vi "InsertDBNew.vi"(9 "String":string, 11 "Entity":string) -> (0 "error out":errorcluster)   [LabVIEW 2012]
uses:
  Global1.vi
  <vilib>/addons/database/Connection.llb/DB Tools Open Connec (Path).vi
  <vilib>/Utility/file.llb/Read From Spreadsheet File (string).vi
  <vilib>/Utility/file.llb/Read From Spreadsheet File (I64).vi
  <vilib>/addons/database/Connection.llb/Conn Execute.vi
  <vilib>/addons/database/Recordset.llb/Rec Fetch Integer Data (R).vi
  <vilib>/addons/database/Recordset.llb/Rec Destroy - Connection.vi
  <vilib>/regexp/Match Regular Expression.xnode
  <vilib>/addons/database/NI_Database_API.lvlib
panel:
  out "output cluster":T1
  out "PathM100":path=path "c:/m100"
  out "appended path":path
  out "concatenated string":string
  out "file or folder exists?":bool
  out "element 7":string
  out "before substring 9":string
  in  "input cluster":T1
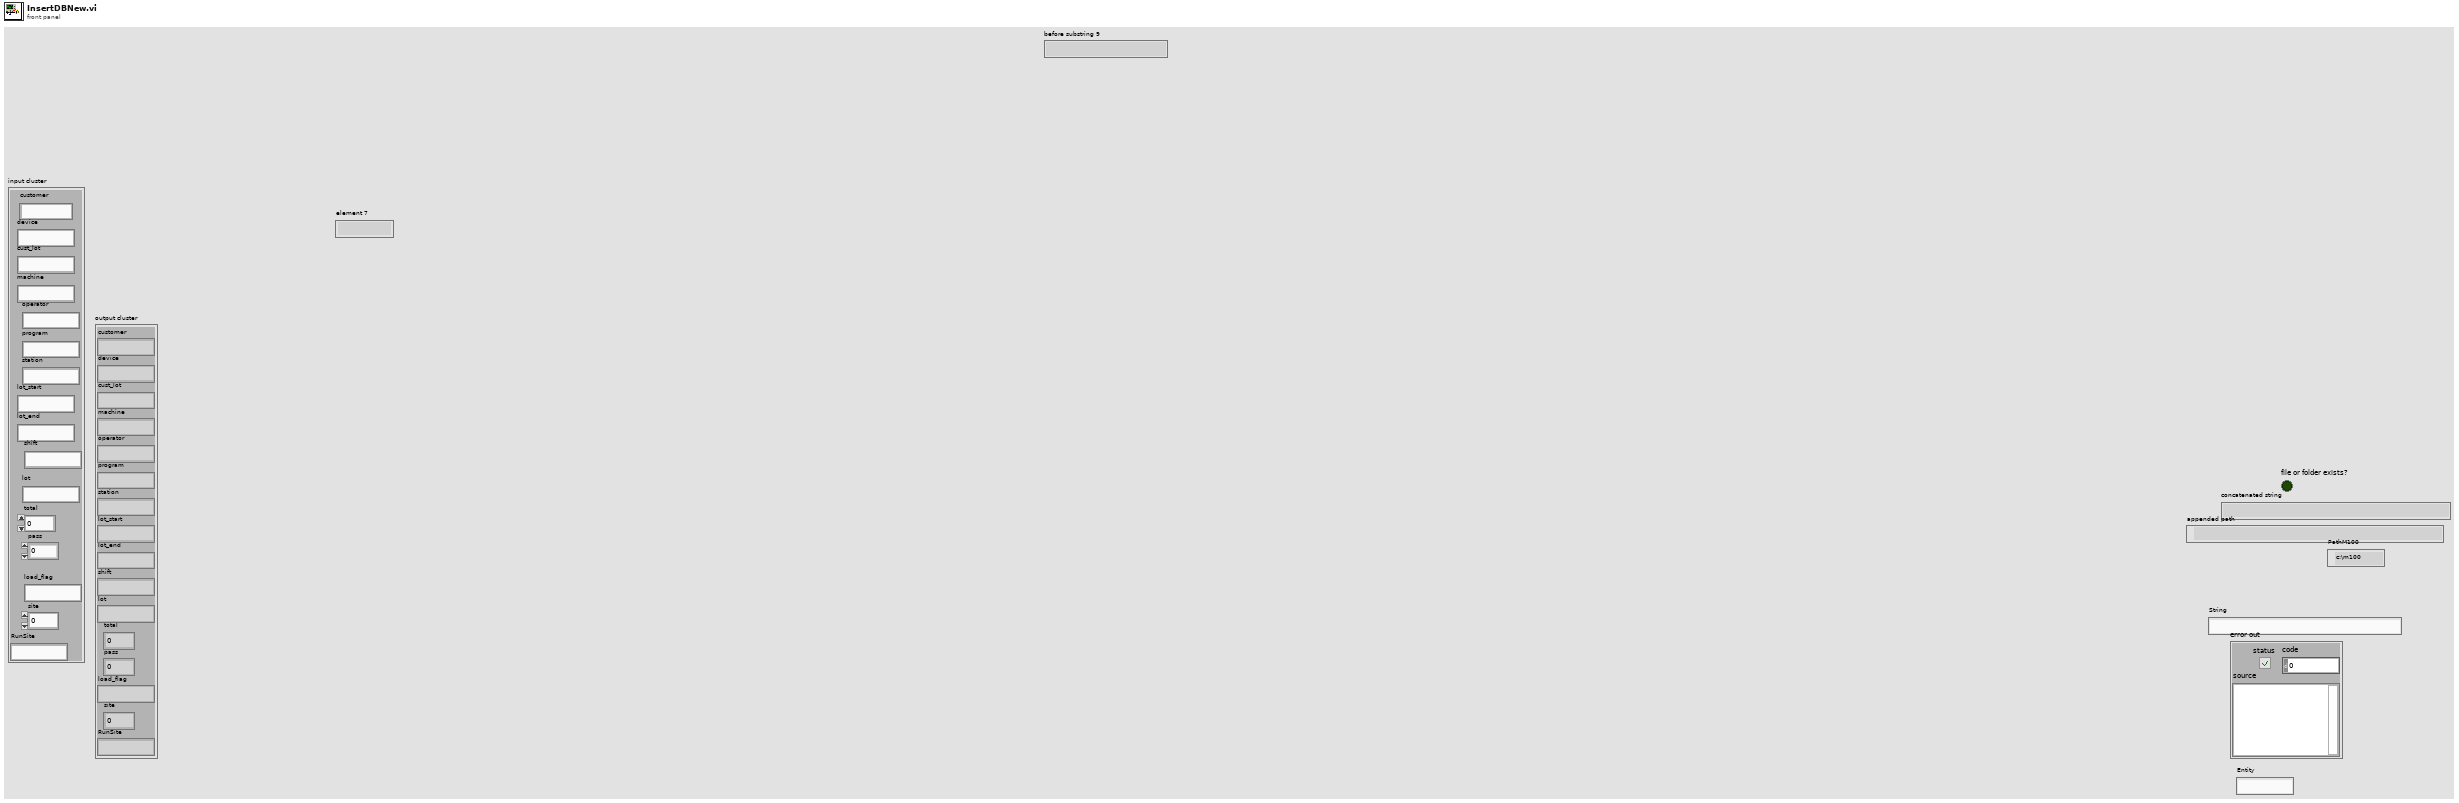
[diagram p1: front panel]
types:
  T1 = cluster{"customer":string, "device":string, "cust_lot":string, "machine":string, "operator":string, "program":string, "station":string, "lot_start":string, "lot_end":string, "shift":string, "lot":string, "total":dbl, "pass":dbl, "load_flag":string, "site":dbl, "RunSite":string}
  T2 = typedef "NI_Database_API.lvlib/Conn ObjectReference.ctl" = refnum<k1>
  T3 = typedef "NI_Database_API.lvlib/Rec ObjectReference.ctl" = refnum<k1>
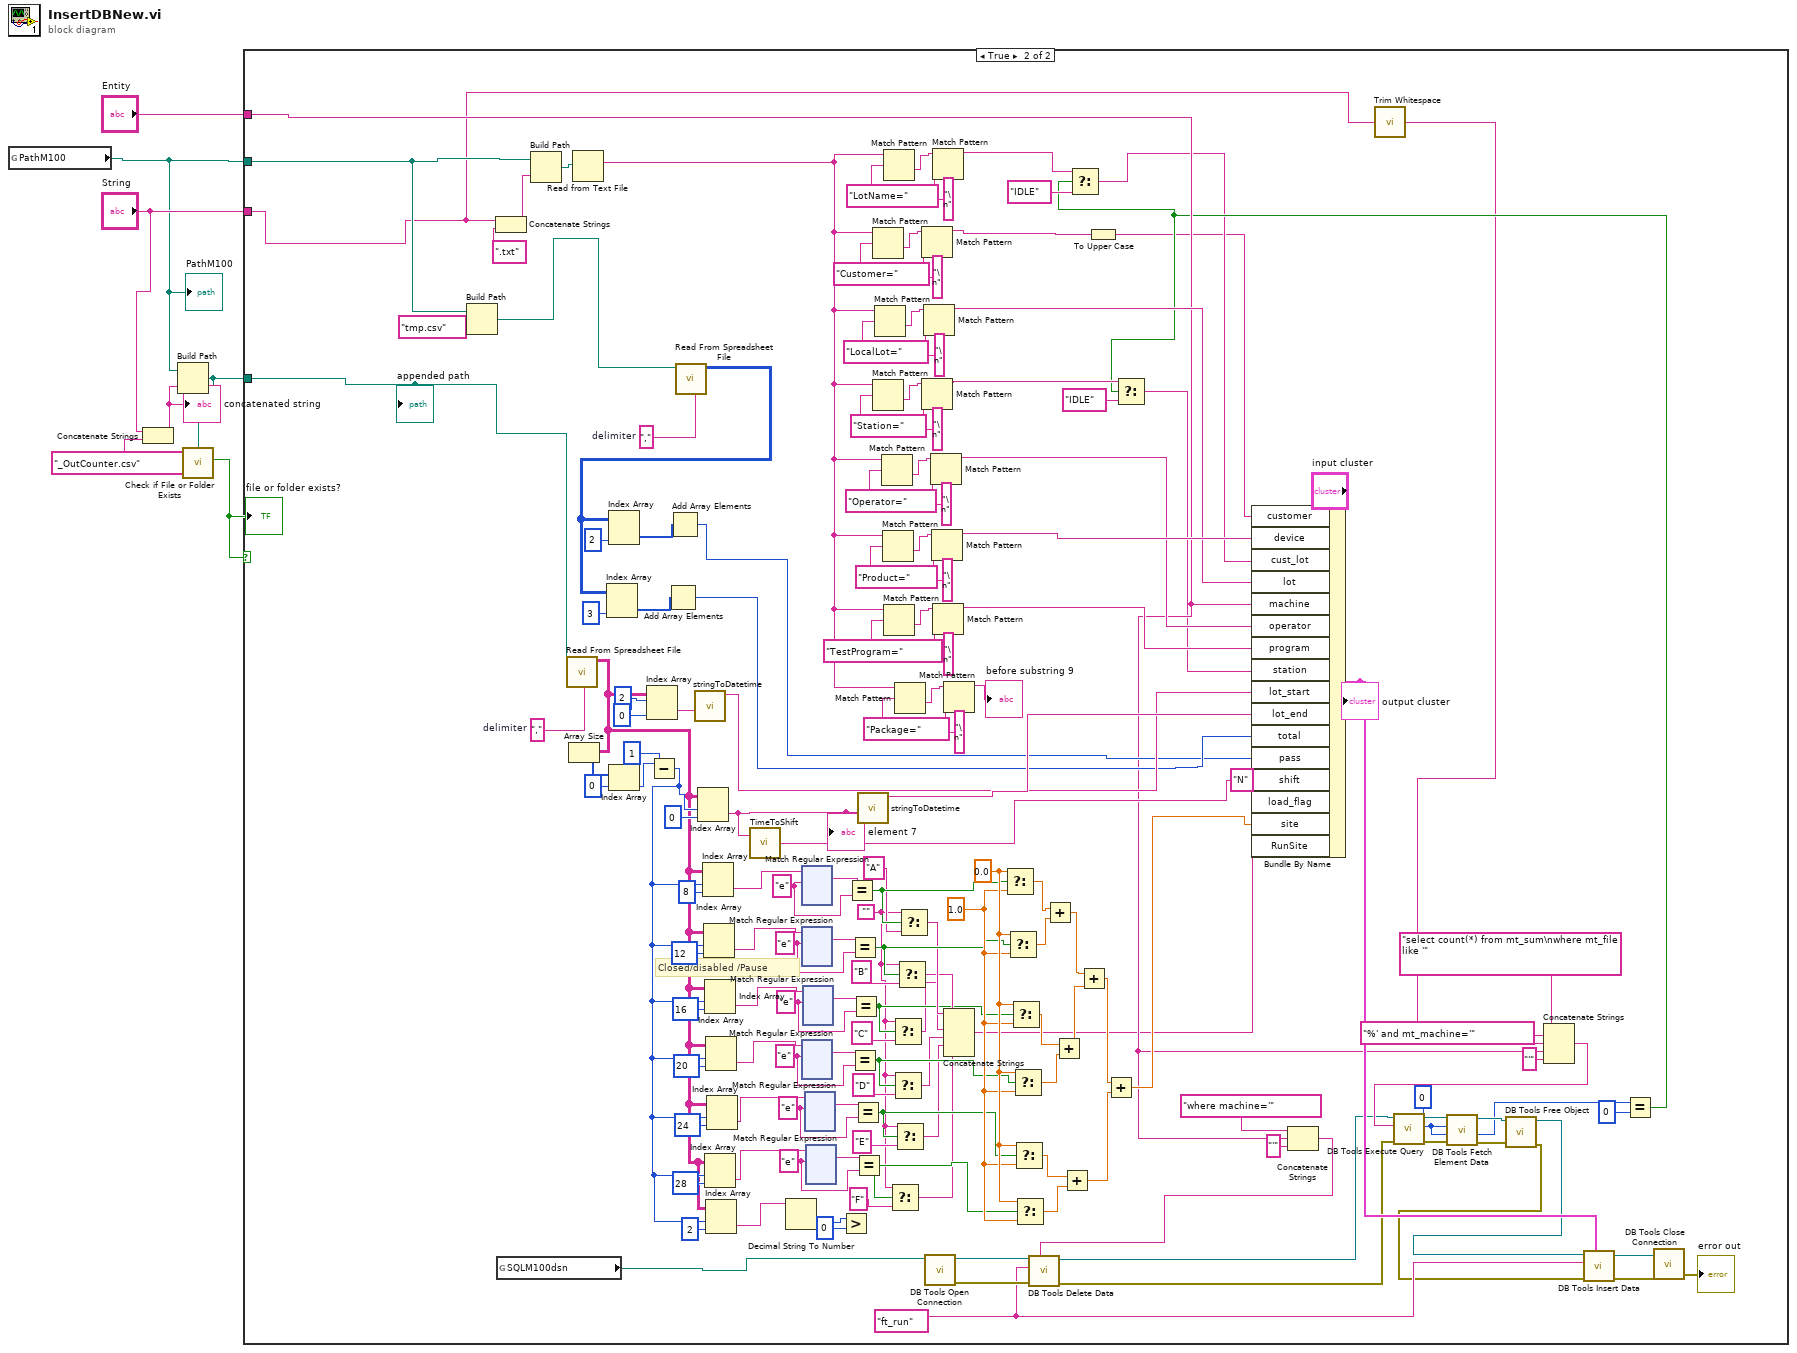
[diagram p0: block diagram]
diagram:
  n1 = global read "Global1.vi" "PathM100"() -> (w1:path)
  "PathM100" <- w1
  n2 = Concatenate Strings("String", "_OutCounter.csv" ("string")) -> (w5:string)
  "concatenated string" <- w5
  n3 = Build Path(base path=w1, name or relative path=w5) -> (appended path=w4:path)
  n4 = call <vilib>:"Check if File or Folder Exists.vi"("path"=w4) -> ("file or folder exists?"=w3:bool)  [unwired: 8 in, 2 out]
  "file or folder exists?" <- w3
  n5 = case shown="True" w3 {
    tunnel: "Entity" -> [_ w39]
    tunnel: "String" -> [_ w31]
    tunnel: w1 -> [_ w168]
    tunnel: w4 -> [_ w167]
    frame False {
    }
    frame True {
      w12 = ""
      w45 = 0
      w72 = 1.0 ("f")
      w73 = 0.0 ("t")
      w92 = "e" ("regular expression")
      w94 = "e" ("regular expression")
      w96 = "e" ("regular expression")
      w98 = "e" ("regular expression")
      w100 = "e" ("regular expression")
      w102 = "e" ("regular expression")
      w126 = ","  # delimiter
      w62 = "ft_run" ("table")
      w137 = ","  # delimiter
      # "Closed/disabled /Pause"
      n6 = Build Path(base path=w168, name or relative path="tmp.csv") -> (appended path=w117:path)
      n7 = Concatenate Strings(w31, ".txt" ("string")) -> (w166:string)
      n8 = global read "Global1.vi" "SQLM100dsn"() -> (w65:path)
      n9 = Build Path(base path=w168, name or relative path=w166) -> (appended path=w163:path)
      n10 = call-poly <vilib>:"Read From Spreadsheet File.vi"("delimiter (\\t)"=w126, "file path (dialog if empty)"=w167) -> ("all rows"=w69:string[][])  [unwired: 5 in, 4 out]
      n11 = Array Size(array=w69) -> (size(s)=w122:i32[])
      n12 = Read from Text File(file (use dialog)=w163) -> (text=w138:string)  [unwired: 3 in, 3 out]
      n13 = Index Array(array=w122, index=0) -> (element=w120:i32)
      n14 = Index Array(array=w69, index (row)=2 ("disabled index (row)"), index (col)=0 ("disabled index (col)")) -> (element=w123:string)
      n15 = Subtract(x=w120, y=1) -> (x-y=w71:i32)
      n16 = call-poly <vilib>:"Read From Spreadsheet File.vi"("delimiter (\\t)"=w137, "file path (dialog if empty)"=w117) -> ("all rows"=w132:i64[][])  [unwired: 5 in, 4 out]
      n17 = Index Array(array=w132, index (col)=3 ("disabled index (col)")) -> (element=w133:i64[])  [unwired: 1 in]
      n18 = Index Array "Index Array"(array=w132, index (col)=2 ("disabled index (col)")) -> (element=w135:i64[])  [unwired: 1 in]
      n19 = Add Array Elements(numeric array=w133) -> (sum=w41:i64)
      n20 = Add Array Elements(numeric array=w135) -> (sum=w40:i64)
      n21 = call "stringToDatetime.vi"("input string"=w123) -> ("sqltime string"=w57:string)  [unwired: 7 in, 3 out]
      n22 = Index Array(array=w69, index (row)=w71, index (col)=0 ("disabled index (col)")) -> (element=w114:string)
      "element 7" <- w114
      n23 = Index Array(array=w69, index (row)=w71, index (col)=8 ("disabled index (col)")) -> (element=w86:string)
      n24 = Index Array(array=w69, index (row)=w71, index (col)=12 ("disabled index (col)")) -> (element=w87:string)
      n25 = Index Array(array=w69, index (row)=w71, index (col)=16 ("disabled index (col)")) -> (element=w88:string)
      n26 = Index Array(array=w69, index (row)=w71, index (col)=28 ("disabled index (col)")) -> (element=w91:string)
      n27 = Index Array(array=w69, index (row)=w71, index (col)=20 ("disabled index (col)")) -> (element=w89:string)
      n28 = Index Array(array=w69, index (row)=w71, index (col)=2) -> (element=w68:string)
      n29 = Index Array(array=w69, index (row)=w71, index (col)=24 ("disabled index (col)")) -> (element=w90:string)
      n30 = call "TimeToShift.vi"("input string"=w114) -> ("s? t:f"=w115:string)  [unwired: 1 in]
      n31 = Decimal String To Number(string=w68) -> (number=w67:i32)  [unwired: 2 in, 1 out]
      n32 = xnode "Match Regular Expression"("input string"=w86, "regular expression"=w102) -> ("whole match"=w103:string)  [unwired: 4 in, 4 out]
      n33 = xnode "Match Regular Expression"("input string"=w87, "regular expression"=w100) -> ("whole match"=w101:string)  [unwired: 4 in, 4 out]
      n34 = xnode "Match Regular Expression"("input string"=w89, "regular expression"=w96) -> ("whole match"=w97:string)  [unwired: 4 in, 4 out]
      n35 = xnode "Match Regular Expression"("input string"=w88, "regular expression"=w98) -> ("whole match"=w99:string)  [unwired: 4 in, 4 out]
      n36 = xnode "Match Regular Expression"("input string"=w90, "regular expression"=w94) -> ("whole match"=w95:string)  [unwired: 4 in, 4 out]
      n37 = xnode "Match Regular Expression"("input string"=w91, "regular expression"=w92) -> ("whole match"=w93:string)  [unwired: 4 in, 4 out]
      n38 = Greater?(x=w67, y=0) -> ()  [unwired: 1 out]
      n39 = Equal?(x=w103, y=w102) -> (x = y?=w29:bool)
      n40 = Equal?(x=w101, y=w100) -> (x = y?=w28:bool)
      n41 = Equal?(x=w97, y=w96) -> (x = y?=w23:bool)
      n42 = Equal?(x=w99, y=w98) -> (x = y?=w25:bool)
      n43 = Equal?(x=w95, y=w94) -> (x = y?=w22:bool)
      n44 = Equal?(x=w93, y=w92) -> (x = y?=w21:bool)
      n45 = call "stringToDatetime.vi"("input string"=w114) -> ("sqltime string"=w58:string)  [unwired: 7 in, 3 out]
      n46 = Match Pattern(string=w138, regular expression="Customer=") -> (after substring=w159:string)  [unwired: 1 in, 3 out]
      n47 = Match Pattern(string=w138, regular expression="Station=") -> (after substring=w153:string)  [unwired: 1 in, 3 out]
      n48 = Match Pattern(string=w138, regular expression="LocalLot=") -> (after substring=w156:string)  [unwired: 1 in, 3 out]
      n49 = Match Pattern(string=w138, regular expression="Operator=") -> (after substring=w150:string)  [unwired: 1 in, 3 out]
      n50 = Match Pattern(string=w138, regular expression="Product=") -> (after substring=w147:string)  [unwired: 1 in, 3 out]
      n51 = Match Pattern(string=w138, regular expression="LotName=") -> (after substring=w162:string)  [unwired: 1 in, 3 out]
      n52 = Match Pattern(string=w138, regular expression="TestProgram=") -> (after substring=w144:string)  [unwired: 1 in, 3 out]
      n53 = Select(t=w12, s=w21, f="F" ("t")) -> (s? t:f=w18:string)
      n54 = Select(t=w12, s=w25, f="C" ("t")) -> (s? t:f=w24:string)
      n55 = Select(t=w12, s=w23, f="D" ("t")) -> (s? t:f=w20:string)
      n56 = Match Pattern(string=w138, regular expression="Package=") -> (after substring=w141:string)  [unwired: 1 in, 3 out]
      n57 = Select(t=w12, s=w22, f="E" ("t")) -> (s? t:f=w19:string)
      n58 = Select(t=w12, s=w28, f="B" ("t")) -> (s? t:f=w26:string)
      n59 = Select(t=w12, s=w29, f="A") -> (s? t:f=w27:string)
      n60 = Match Pattern(string=w159, regular expression="\n") -> (before substring=w9:string)  [unwired: 1 in, 3 out]
      n61 = Match Pattern(string=w153, regular expression="\n") -> (before substring=w42:string)  [unwired: 1 in, 3 out]
      n62 = Match Pattern(string=w156, regular expression="\n") -> (before substring=w129:string)  [unwired: 1 in, 3 out]
      n63 = call-poly <vilib>:"DB Tools Open Connection.vi"("connection information"=w65) -> ("error out"=w63:errorcluster, "connection reference"=w64:T2)  [unwired: 7 in]
      n64 = Match Pattern(string=w150, regular expression="\n") -> (before substring=w128:string)  [unwired: 1 in, 3 out]
      n65 = Match Pattern(string=w147, regular expression="\n") -> (before substring=w130:string)  [unwired: 1 in, 3 out]
      n66 = Match Pattern(string=w162, regular expression="\n") -> (before substring=w33:string)  [unwired: 1 in, 3 out]
      n67 = Match Pattern(string=w144, regular expression="\n") -> (before substring=w127:string)  [unwired: 1 in, 3 out]
      n68 = Match Pattern(string=w141, regular expression="\n") -> (before substring=→"before substring 9":string)  [unwired: 1 in, 3 out]
      n69 = Concatenate Strings(w27, w26, w24, w20, w19, w18) -> (w10:string)
      n70 = Select(t=w73, s=w29, f=w72) -> (s? t:f=w84:dbl)
      n71 = Select(t=w73, s=w28, f=w72) -> (s? t:f=w85:dbl)
      n72 = Select(t=w73, s=w25, f=w72) -> (s? t:f=w83:dbl)
      n73 = Select(t=w73, s=w23, f=w72) -> (s? t:f=w82:dbl)
      n74 = Select(t=w73, s=w22, f=w72) -> (s? t:f=w81:dbl)
      n75 = Select(t=w73, s=w21, f=w72) -> (s? t:f=w80:dbl)
      n76 = Add(x=w84, y=w85) -> (x+y=w78:dbl)
      n77 = Add(x=w83, y=w82) -> (x+y=w79:dbl)
      n78 = Add(x=w81, y=w80) -> (x+y=w77:dbl)
      n79 = Add(x=w78, y=w79) -> (x+y=w76:dbl)
      n80 = To Upper Case(1:w9) -> (0:w8:string)
      n81 = Add(x=w76, y=w77) -> (x+y=w75:dbl)
      n82 = Concatenate Strings("where machine='" ("string"), w39, "'" ("string")) -> (w59:string)
      n83 = call <vilib>:"DB Tools Delete Data.vi"("condition"=w59, "error in (no error)"=w63, "table"=w62, "connection reference"=w64) -> ("error out"=w48:errorcluster, "connection reference out"=w49:T2)  [unwired: 6 in]
      n84 = call <vilib>:"Trim Whitespace.vi"("string"=w31) -> ("trimmed string"=w30:string)  [unwired: 1 in]
      n85 = Concatenate Strings("select count(*) from mt_sum\nwhere mt_file like '", w30, "%' and mt_machine='" ("string"), w39, "'" ("string")) -> (w50:string)
      n86 = call-poly <vilib>:"DB Tools Execute Query.vi"("error in (no error)"=w48, "SQL query"=w50, "connection reference"=w49) -> ("error out"=w54:errorcluster, "recordset reference"=w53:T3)  [unwired: 5 in]
      n87 = call-poly <vilib>:"DB Tools Fetch Element Data.vi"("error in (no error)"=w54, "type"=w45, "column index"=w45, "recordset reference"=w53) -> ("error out"=w52:errorcluster, "data"=w44:i32, "recordset reference out"=w51:T3)  [unwired: 3 in]
      n88 = call-poly <vilib>:"DB Tools Free Object.vi"("error in (no error)"=w52, "recordset reference"=w51) -> ("error out"=w46:errorcluster, "connection reference"=w47:T2)  [unwired: 8 in]
      n89 = Equal?(x=w44, y=0) -> (x = y?=w34:bool)
      n90 = Select(t=w33, s=w34, f="IDLE") -> (s? t:f=w32:string)
      n91 = Select(t=w42, s=w34, f="IDLE") -> (s? t:f=w37:string)
      n92 = Bundle By Name(cluster="input cluster", "customer"=w8, "device"=w130, "cust_lot"=w32, "lot"=w129, "machine"=w39, "operator"=w128, "program"=w127, "station"=w37, "lot_start"=w57, "lot_end"=w58, "total"=w41, "pass"=w40, "shift"=w115, "load_flag"="N", "site"=w75, "RunSite"=w10) -> (w74:T1)
      "output cluster" <- w74
      n93 = call <vilib>:"DB Tools Insert Data.vi"("data"=w74, "error in (no error)"=w46, "table"=w62, "connection reference"=w47) -> ("error out"=w112:errorcluster, "connection reference out"=w113:T2)  [unwired: 6 in]
      n94 = call <vilib>:"DB Tools Close Connection.vi"("error in (no error)"=w112, "connection reference"=w113) -> ("error out"=→"error out":errorcluster)  [unwired: 5 in]
      "appended path" <- w167
    }
  }
